vi "ReadParse_SubVI.vi"(3 "error in (no error)":errorcluster) -> (7 "Read Results":T1, 10 "error out":errorcluster)   [LabVIEW 2017]
uses:
  TCP_Read_Enum.ctl
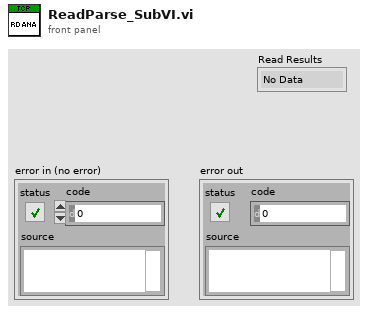
[diagram p1: front panel]
types:
  T1 = typedef "TCP_Read_Enum.ctl" = enum16{"No Data", "New Data", "No Connection"}
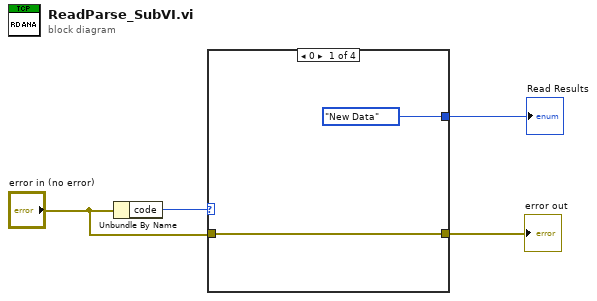
[diagram p0: block diagram]
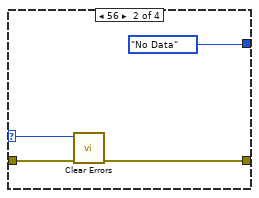
[diagram p2: hidden frame]
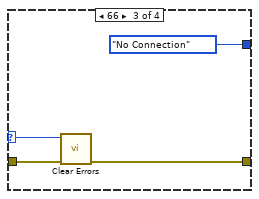
[diagram p3: hidden frame]
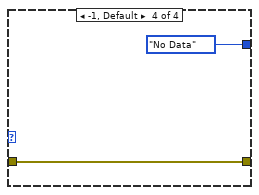
[diagram p4: hidden frame]
diagram:
  n1 = Unbundle By Name("error in (no error)") -> ("code"=w4:i32)
  n2 = case shown="0" w4 {
    selector: w4 -> [_ w9 w12 _]
    tunnel: "error in (no error)" -> [w6 w8 w13 w16]
    tunnel: [w6 w7 w11 w16] -> w2
    tunnel: [TCP_Read_Enum."New Data" ("Enum") TCP_Read_Enum."No Data" ("Enum") TCP_Read_Enum."No Connection" ("Enum") TCP_Read_Enum."No Data" ("Enum")] -> w1
    frame 0 {
    }
    frame 56 {
      n3 = call <vilib>:"Clear Errors.vi"("error in (no error)"=w8, "specific error code to clear (0: all)"=w9) -> ("error out"=w7:errorcluster)  [unwired: 4 in, 1 out]
    }
    frame 66 {
      n4 = call <vilib>:"Clear Errors.vi"("error in (no error)"=w13, "specific error code to clear (0: all)"=w12) -> ("error out"=w11:errorcluster)  [unwired: 4 in, 1 out]
    }
    frame -1, Default {
    }
  }
  "error out" <- w2
  "Read Results" <- w1
